vi "ImportLog.vi"(8 "error in (no error)":errorcluster, 11 "Missing Variables":string[](array[string])) -> (0 "error out":errorcluster)   [LabVIEW 2017, in "Shared Variables CD 2.0 Configuration.lvlib"]
uses:
  Shared Variables CD 2.0 Configuration.lvlib
panel:
  out "Missing Variables 2":string[](array[string])
  in  "Write to File 3":bool
  in  "Exit":bool
  in  "Write to File":bool
  # "Missing or unreachable shared variables"
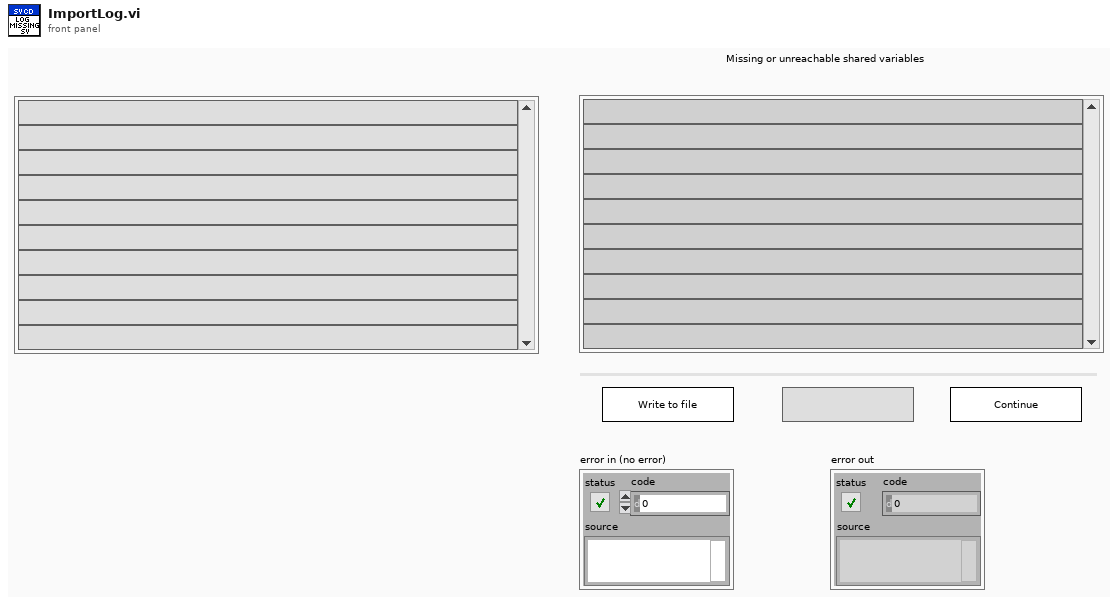
[diagram p1: front panel]
types:
  T1 = enum32{"Invalid", "Standard", "Closed", "Hidden", "Minimized", "Maximized"}
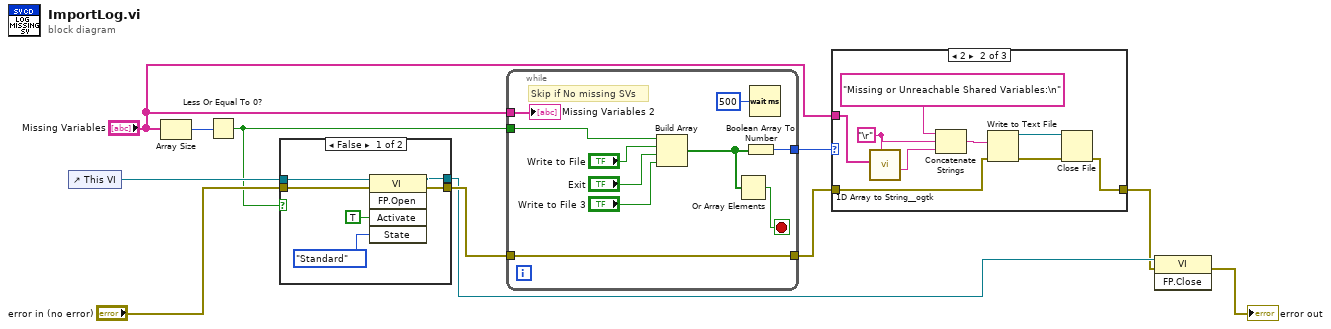
[diagram p0: block diagram]
diagram:
  n1 = control-ref of="This VI"() -> (w9:refnum<vi>)
  n2 = Array Size(array="Missing Variables") -> (size(s)=w11:i32)
  n3 = Less Or Equal To 0?(x=w11) -> (x <= 0?=w2:bool)
  n4 = case shown="False" w2 {
    tunnel: w9 -> [w17 w19]
    tunnel: "error in (no error)" -> [w16 w18]
    tunnel: [w15 w18] -> w7
    tunnel: [w13 w19] -> w5
    frame False {
      n5 = invoke class="VI" method="FP.Open"(reference=w17, error in=w16, "Activate"=TRUE ("Activate?"), "State"=T1."Standard") -> (reference out=w13:refnum<vi>, error out=w15:errorcluster)  [unwired: 1 in, 3 out]
    }
    frame True {
    }
  }
  n6 = while {
    tunnel: [w27] -> w10
    tunnel: w2 -> [w22]
    tunnel: w7 -> [w21]
    tunnel: [w21] -> w4
    tunnel: "Missing Variables" -> [w20]
    stop <- w25 stop-if-true
    # "Skip if No missing SVs"
    n7 = Build Array(w22, "Write to File", "Exit", "Write to File 3") -> (w24:bool[])
    n8 = Or Array Elements(Boolean array=w24) -> (logical OR=w25:bool)
    n9 = Boolean Array To Number(Boolean array=w24) -> (number=w27:u32)
    n10 = Wait (ms)(milliseconds to wait=u32 500) -> ()  [unwired: 1 out]
    "Missing Variables 2" <- w20
  }
  n11 = case shown="2" w10 {
    tunnel: "Missing Variables" -> [_ w39 _]
    tunnel: w4 -> [w30 w35 w40]
    tunnel: [w30 w33 w40] -> w3
    frame 0, Default {
    }
    frame 2 {
      w31 = "\r"
      n12 = call <userlib>:"1D Array to String__ogtk.vi"("delimiter (Tab)"=w31, "Array of Strings"=w39) -> ("delimited string"=w32:string)  [unwired: 9 in]
      n13 = Concatenate Strings("Missing or Unreachable Shared Variables:\n" ("string"), w31, w32) -> (w37:string)
      n14 = Write to Text File(text=w37, error in=w35) -> (refnum out=w36:refnum<file>, error out=w34:errorcluster)  [unwired: 2 in, 1 out]
      n15 = Close File(refnum=w36, error in=w34) -> (error out=w33:errorcluster)  [unwired: 1 out]
    }
    frame 4 {
    }
  }
  n16 = invoke class="VI" method="FP.Close"(reference=w5, error in=w3) -> (error out=→"error out":errorcluster)  [unwired: 1 in, 2 out]
